vi "SIMULATION_SIM_MODULE_EXECUTE.vi"(6 "FPGA_Time_Seconds":dbl=-1.0, 7 "Module Index":i32, 8 "error in (no error)":errorcluster, 9 "Battery Voltage":dbl) -> (0 "error out":errorcluster, 1 "current":dbl, 2 "Swerve Distance_Radians":dbl, 3 "Wheel Distance_Meters":dbl)   [LabVIEW 2019]
uses:
  <vilib>/Rock Robotics/WPI/ThirdParty/JAS_Junk/TrajLib/Enum/DCMOTOR_TYPES_ENUM.ctl
  <vilib>/Rock Robotics/WPI/ThirdParty/JAS_Junk/TrajLib/VI/Util_GetTime_U32.vi
  SIMULATION_SIM_Globals.vi
  <vilib>/Rock Robotics/WPI/ThirdParty/JAS_Junk/TrajLib/VI/Util_GetTime_U64.vi
  <vilib>/Rock Robotics/WPI/ThirdParty/JAS_Junk/TrajLib/Trajectory_Library.lvlib
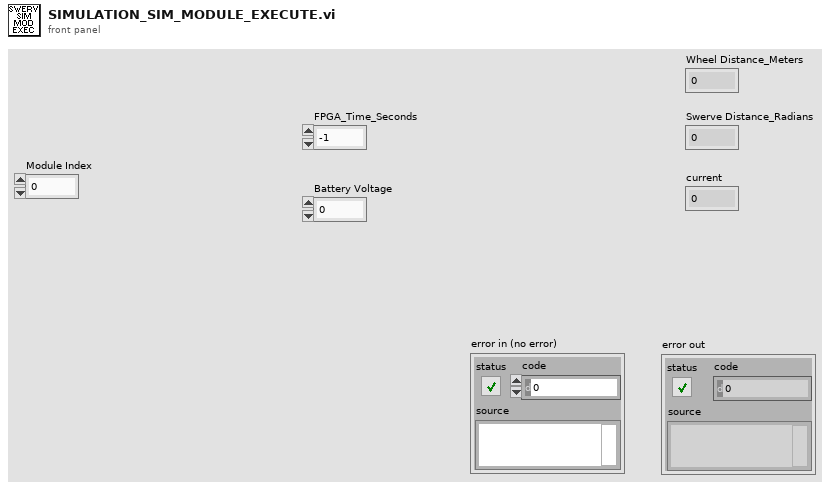
[diagram p1: front panel]
types:
  T1 = typedef "Trajectory_Library.lvlib/DCMOTOR_TYPES_ENUM.ctl" = enum16{"CIM", "AndyMark 9015", "Andy Mark RS 775 125", "Bag", "BaneBots RS 550", "BaneBots RS 775", "Falcon 500", "Mini CIM", "NEO", "NEO 550", "Romi BuiltIn", "Vex 775 Pro", "Snow Blower AM 2235A", "Bosch Seat AM 3493"}
  T2 = cluster{"Swerve Motor Device Index":i32, "Drive Motor Device Index":i32, "Swerve Encoder Device Index":i32, "Drive Encoder Device Index":i32, "Drive DistPerzcount":dbl, "SwerveRadPerCount":dbl}[]
  T3 = cluster{"Swerve Motor Device Index":i32, "Drive Motor Device Index":i32, "Swerve Encoder Device Index":i32, "Drive Encoder Device Index":i32, "Drive DistPerzcount":dbl, "SwerveRadPerCount":dbl}
  T4 = typedef "Trajectory_Library.lvlib/LINEAR_SYSTEM_ID_DCMOTOR_MODEL.ctl" = cluster{"DCMOTOR_TYPES":T1, "Num Motors":i32, "Gearing":dbl, "MOI kgm2":dbl}
  T5 = typedef "Trajectory_Library.lvlib/DCMOTOR_SIM_SIMULATION_PARAMS.ctl" = cluster{"Pos Sim Std Dev Rotations":dbl, "Vel Sim Std Dev RPM":dbl}
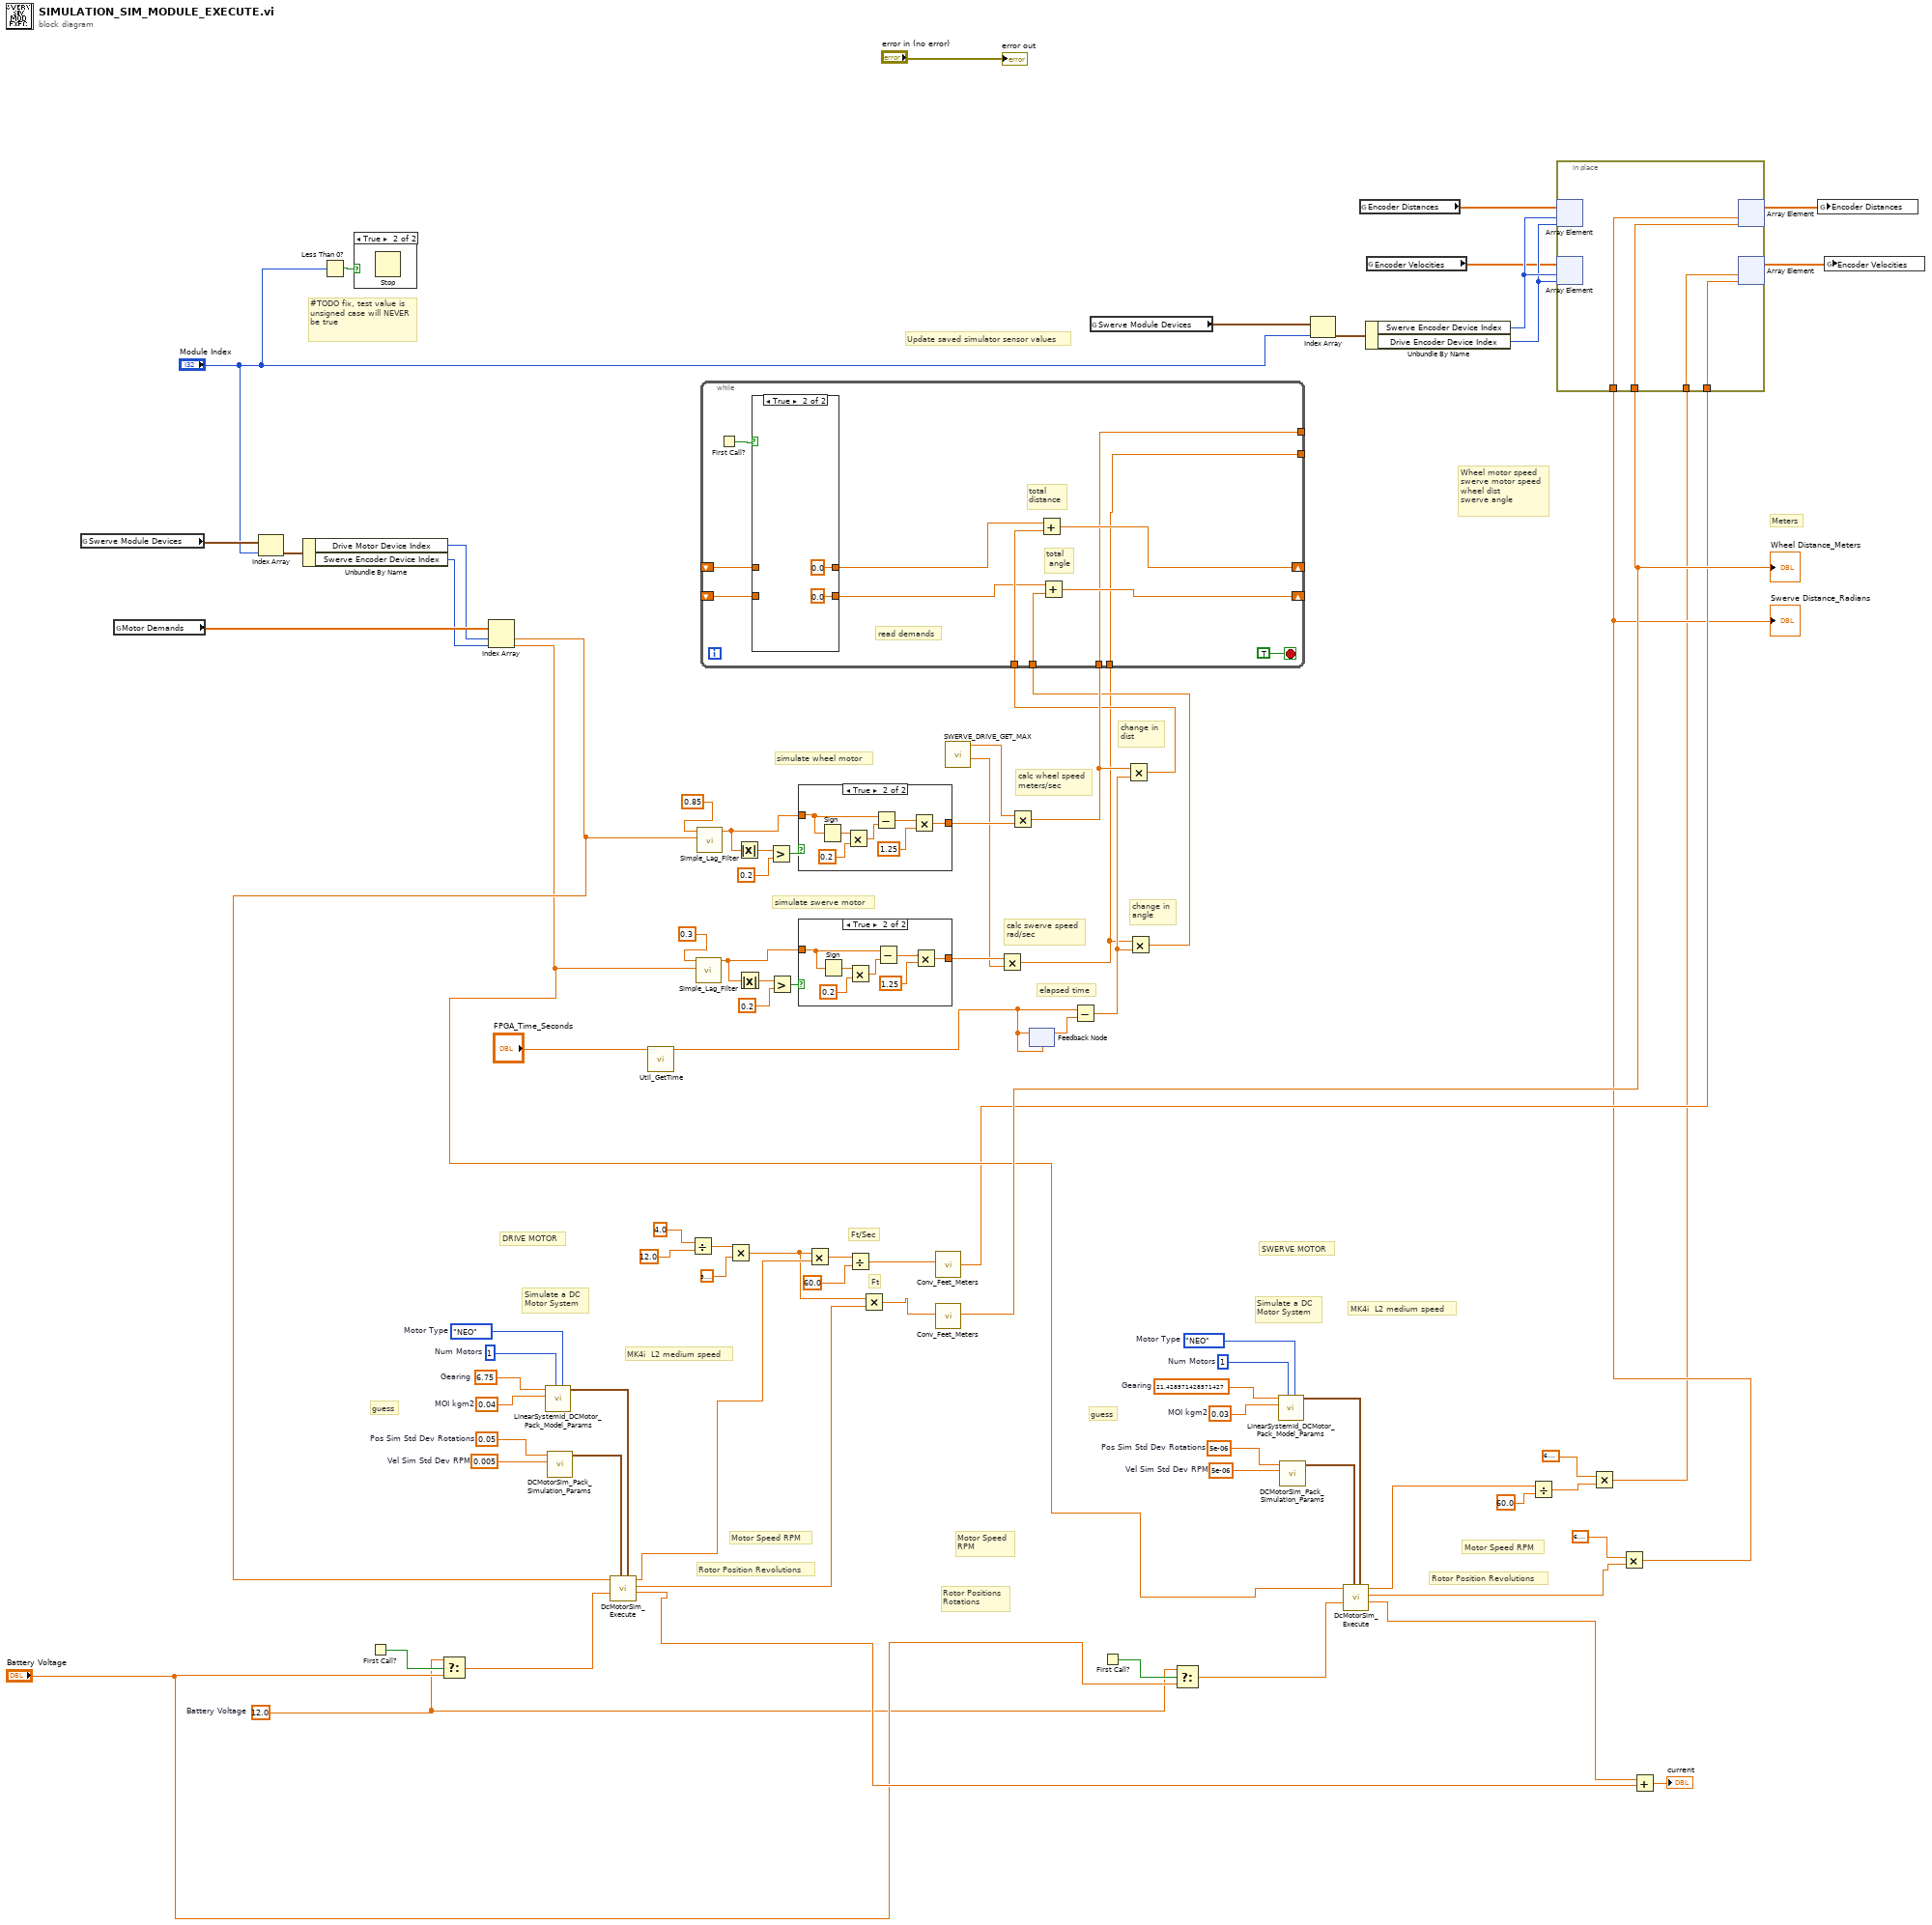
[diagram p0: block diagram]
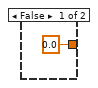
[diagram p3: hidden frame]
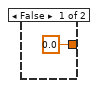
[diagram p4: hidden frame]
diagram:
  w27 = 0.05  # Pos Sim Std Dev Rotations
  w28 = 0.005  # Vel Sim Std Dev RPM
  w31 = 6.75  # Gearing
  w32 = 0.04  # MOI kgm2
  w33 = 1  # Num Motors
  w34 = DCMOTOR_TYPES_ENUM."NEO"  # Motor Type
  w37 = 5e-06  # Pos Sim Std Dev Rotations
  w38 = 5e-06  # Vel Sim Std Dev RPM
  w41 = 21.428571428571427  # Gearing
  w42 = 0.03  # MOI kgm2
  w43 = 1  # Num Motors
  w44 = DCMOTOR_TYPES_ENUM."NEO"  # Motor Type
  w24 = 12.0  # Battery Voltage
  # "guess"
  # "guess"
  # "Ft/Sec"
  # "Ft"
  # "MK4i  L2 medium speed"
  # "MK4i  L2 medium speed"
  # "Rotor Position Revolutions"
  # "Motor Speed RPM"
  # "Simulate a DC \nMotor System"
  # "Rotor Position Revolutions"
  # "Motor Speed RPM"
  # "Simulate a DC \nMotor System"
  # "SWERVE MOTOR"
  # "DRIVE MOTOR"
  # "Rotor Positions\nRotations"
  # "Motor Speed\nRPM"
  # "Update saved simulator sensor values"
  # "Wheel motor speed\nswerve motor speed\nwheel dist\nswerve angle"
  # "change in\nangle"
  # "change in\ndist"
  # "calc wheel speed\nmeters/sec"
  # "calc swerve speed\nrad/sec"
  # "simulate swerve motor"
  # "simulate wheel motor"
  # "#TODO fix, test value is unsigned case will NEVER be true"
  # "elapsed time"
  # "Meters"
  n1 = global read "SIMULATION_SIM_Globals.vi" "Swerve Module Devices"() -> (w55:T2)
  n2 = global read "SIMULATION_SIM_Globals.vi" "Motor Demands"() -> (w53:dbl[])
  n3 = Index Array(array=w55, index="Module Index") -> (element=w54:T3)
  n4 = Unbundle By Name(w54) -> ("Drive Motor Device Index"=w52:i32, "Swerve Encoder Device Index"=w51:i32)
  n5 = Less Than 0?(x="Module Index") -> (x < 0?=w83:bool)
  n6 = case shown="True" w83 {
    frame False {
    }
    frame True {
      n7 = Stop() -> ()  [unwired: 1 in]
    }
  }
  n8 = First Call?() -> (First Call?: T/F=w25:bool)
  n9 = Select(t=w24, s=w25, f="Battery Voltage") -> (s? t:f=w26:dbl)
  n10 = Index Array(array=w53, index #1=w52, index #2=w51) -> (element #1=w49:dbl, element #2=w5:dbl)
  n11 = call <vilib>:"LinearSystemId_DCMotor_Pack_Model_Params.vi"("DCMOTOR_TYPES"=w34, "Num Motors"=w33, "MOI kgm2"=w32, "Gearing"=w31) -> ("LinearSystem_ID_DCMotor_Model"=w30:T4)  [unwired: 7 in]
  n12 = call <vilib>:"DCMotorSim_Pack_Simulation_Params.vi"("Vel Sim Std Dev RPM"=w28, "Pos Sim Std Dev Rotations"=w27) -> ("DCMOTOR_Sim_Simulation_Params"=w29:T5)  [unwired: 9 in]
  n13 = call <vilib>:"DcMotorSim_Execute.vi"("DCMotor_Model _Params"=w30, "DCMOTORSim_Simulation_Params"=w29, "Battery Voltage"=w26, "Motor Dmd (CO)"=w49) -> ("Motor Current"=w47:dbl, "Position_Rotations"=w17:dbl, "Velocity_RPM"=w19:dbl)  [unwired: 3 in, 2 out]
  n14 = call <vilib>:"Util_GetTime.vi"("Pass_Through_Time"="FPGA_Time_Seconds") -> ("FPGA_Time_Seconds"=w63:dbl)  [unwired: 8 in, 2 out]
  n15 = Divide(x=4.0, y=12.0) -> (x/y=w21:dbl)
  n16 = call "Simple_Lag_Filter.vi"("Input"=w5, "Lag"=0.3) -> ("Lagged Ouptut"=w79:dbl)  [unwired: 9 in]
  n17 = call "Simple_Lag_Filter.vi"("Input"=w49, "Lag"=0.85) -> ("Lagged Ouptut"=w74:dbl)  [unwired: 9 in]
  n18 = Multiply(x=w21, y=3.141592653589793) -> (x*y=w18:dbl)
  n19 = Absolute Value(x=w74) -> (abs(x)=w77:dbl)
  n20 = Absolute Value(x=w79) -> (abs(x)=w82:dbl)
  n21 = Greater?(x=w77, y=0.2) -> (0:w75:bool)
  n22 = Greater?(x=w82, y=0.2) -> (0:w80:bool)
  n23 = case shown="True" w75 {
    tunnel: w74 -> [_ w92]
    tunnel: [0.0 w88] -> w73
    frame False {
    }
    frame True {
      n24 = Sign(1:w92) -> (0:w94:dbl)
      n25 = Multiply(x=w94, y=0.2) -> (x*y=w91:dbl)
      n26 = Subtract(x=w92, y=w91) -> (x-y=w90:dbl)
      n27 = Multiply(x=w90, y=1.25) -> (x*y=w88:dbl)
    }
  }
  n28 = case shown="True" w80 {
    tunnel: w79 -> [_ w100]
    tunnel: [0.0 w96] -> w78
    frame False {
    }
    frame True {
      n29 = Sign(1:w100) -> (0:w102:dbl)
      n30 = Multiply(x=w102, y=0.2) -> (x*y=w99:dbl)
      n31 = Subtract(x=w100, y=w99) -> (x-y=w98:dbl)
      n32 = Multiply(x=w98, y=1.25) -> (x*y=w96:dbl)
    }
  }
  n33 = Multiply(x=w18, y=w19) -> (x*y=w16:dbl)
  n34 = Divide(x=w16, y=60.0) -> (x/y=w14:dbl)
  n35 = Multiply(x=w18, y=w17) -> (x*y=w13:dbl)
  n36 = call <vilib>:"Conv_Feet_Meters.vi"("Feet"=w14) -> ("Meters"=w4:dbl)  [unwired: 10 in]
  n37 = call <vilib>:"Conv_Feet_Meters.vi"("Feet"=w13) -> ("Meters"=w12:dbl)  [unwired: 10 in]
  "Wheel Distance_Meters" <- w12
  n38 = call "SWERVE_DRIVE_GET_MAX.vi"() -> ("Max Rotational Vel (Rad/Sec)"=w69:dbl, "Max Wheel Vel (Meter/Sec)"=w72:dbl)  [unwired: 10 in]
  n39 = Multiply(x=w78, y=w69) -> (x*y=w3:dbl)
  n40 = Multiply(x=w72, y=w73) -> (x*y=w84:dbl)
  n41 = feedback #1(w63) -> (w71:dbl)
  n42 = feedback-in #1(w63) -> ()
  n43 = Subtract(x=w63, y=w71) -> (x-y=w70:dbl)
  n44 = global read "SIMULATION_SIM_Globals.vi" "Swerve Module Devices"() -> (w64:T2)
  n45 = First Call?() -> (First Call?: T/F=w35:bool)
  n46 = Multiply(x=w84, y=w70) -> (x*y=w66:dbl)
  n47 = Multiply(x=w3, y=w70) -> (x*y=w65:dbl)
  n48 = while {
    tunnel: w84 -> [w108]
    tunnel: w3 -> [w107]
    tunnel: w66 -> [w114]
    tunnel: w65 -> [w113]
    shift-right: [w112] -> _
    shift-left: _ -> [w106]
    shift-right: [w111] -> _
    shift-left: _ -> [w104]
    tunnel: [w108] -> _
    tunnel: [w107] -> _
    stop <- TRUE stop-if-true
    # "total \ndistance"
    # "total\n angle"
    # "read demands"
    n49 = First Call?() -> (First Call?: T/F=w109:bool)
    n50 = case shown="True" w109 {
      tunnel: w106 -> [w116 _]
      tunnel: [w116 0.0] -> w105
      tunnel: w104 -> [w115 _]
      tunnel: [w115 0.0] -> w103
      frame False {
      }
      frame True {
      }
    }
    n51 = Add(x=w105, y=w114) -> (x+y=w112:dbl)
    n52 = Add(x=w103, y=w113) -> (x+y=w111:dbl)
  }
  n53 = Select(t=w24, s=w35, f="Battery Voltage") -> (s? t:f=w36:dbl)
  n54 = call <vilib>:"LinearSystemId_DCMotor_Pack_Model_Params.vi"("DCMOTOR_TYPES"=w44, "Num Motors"=w43, "MOI kgm2"=w42, "Gearing"=w41) -> ("LinearSystem_ID_DCMotor_Model"=w40:T4)  [unwired: 7 in]
  n55 = call <vilib>:"DCMotorSim_Pack_Simulation_Params.vi"("Vel Sim Std Dev RPM"=w38, "Pos Sim Std Dev Rotations"=w37) -> ("DCMOTOR_Sim_Simulation_Params"=w39:T5)  [unwired: 9 in]
  n56 = Index Array(array=w64, index="Module Index") -> (element=w62:T3)
  n57 = call <vilib>:"DcMotorSim_Execute.vi"("DCMotor_Model _Params"=w40, "DCMOTORSim_Simulation_Params"=w39, "Battery Voltage"=w36, "Motor Dmd (CO)"=w5) -> ("Motor Current"=w48:dbl, "Position_Rotations"=w6:dbl, "Velocity_RPM"=w10:dbl)  [unwired: 3 in, 2 out]
  n58 = global read "SIMULATION_SIM_Globals.vi" "Encoder Distances"() -> (w59:dbl[])
  n59 = Unbundle By Name(w62) -> ("Swerve Encoder Device Index"=w61:i32, "Drive Encoder Device Index"=w60:i32)
  n60 = global read "SIMULATION_SIM_Globals.vi" "Encoder Velocities"() -> (w58:dbl[])
  n61 = Divide(x=w10, y=60.0) -> (x/y=w9:dbl)
  n62 = Multiply(x=6.283185307179586, y=w9) -> (x*y=w1:dbl)
  n63 = Multiply(x=6.283185307179586, y=w6) -> (x*y=w2:dbl)
  "Swerve Distance_Radians" <- w2
  n64 = in-place {
    in-place-border: w2 -> [w122]
    in-place-border: w12 -> [w121]
    in-place-border: w4 -> [w120]
    in-place-border: w1 -> [w119]
    n65 = in-place-array #2(w59, w61, w60) -> ()  [unwired: 2 out]
    n66 = in-place-array #3(w58, w61, w60) -> ()  [unwired: 2 out]
    n67 = in-place-array #2(w122, w121) -> (w57:dbl[])  [unwired: 2 out]
    n68 = in-place-array #3(w119, w120) -> (w56:dbl[])  [unwired: 2 out]
  }
  n69 = Add(x=w48, y=w47) -> (x+y=→"current":dbl)
  n70 = global write "SIMULATION_SIM_Globals.vi" "Encoder Distances"(w57) -> ()
  n71 = global write "SIMULATION_SIM_Globals.vi" "Encoder Velocities"(w56) -> ()
  "error out" <- "error in (no error)"
